vi "VLC Main Open Camera.vi"(11 "Camera 1":refnum<k24>(container)) -> ()   [LabVIEW 2017]
uses:
  System.Windows.Forms
panel:
  in  "Camera 3":refnum<vi>
  in  "path in":path=path "C:/Program Files (x86)/VideoLAN/VLC/libvlc.dll"
  in  "stop":bool
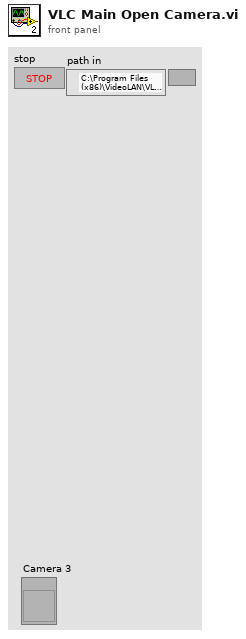
[diagram p1: front panel]
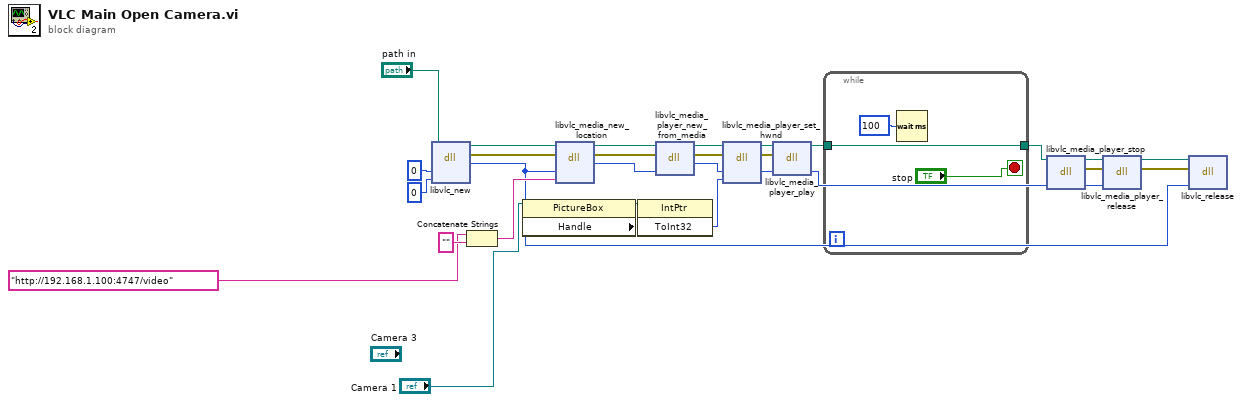
[diagram p0: block diagram]
diagram:
  n1 = dll-call lib="C:/Program Files (x86)/VideoLAN/VLC/libvlc.dll" fn="libvlc_new"(path in="path in", "argc"=i16 0, "argv"=u8 0) -> (path out=w24:path, error out=w21:errorcluster, "return type"=w10:i32)  [unwired: 4 in]
  n2 = Concatenate Strings("http://192.168.1.100:4747/video", "" ("string")) -> (w14:string)
  n3 = property class="PictureBox"(reference="Camera 1") -> ("Handle"=w28:refnum<k24>)  [unwired: 1 in, 2 out]
  n4 = dll-call lib="C:/Program Files (x86)/VideoLAN/VLC/libvlc.dll" fn="libvlc_media_new_location"(path in=w24, error in=w21, "p_instance"=w10, "path"=w14) -> (path out=w27:path, error out=w15:errorcluster, "return type"=w16:i32)  [unwired: 3 in]
  n5 = invoke class="IntPtr" method="ToInt32"(reference=w28) -> ("ToInt32"=w29:i32)  [unwired: 2 in, 2 out]
  n6 = dll-call lib="C:/Program Files (x86)/VideoLAN/VLC/libvlc.dll" fn="libvlc_media_player_new_from_media"(path in=w27, error in=w15, "p_md"=w16) -> (path out=w25:path, error out=w18:errorcluster, "return type"=w20:i32)  [unwired: 2 in]
  n7 = dll-call lib="C:/Program Files (x86)/VideoLAN/VLC/libvlc.dll" fn="libvlc_media_player_set_hwnd"(path in=w25, error in=w18, "p_mi"=w20, "drawable"=w29) -> (path out=w26:path, error out=w17:errorcluster, "p_mi"=w19:i32)  [unwired: 3 in]
  n8 = dll-call lib="C:/Program Files (x86)/VideoLAN/VLC/libvlc.dll" fn="libvlc_media_player_play"(path in=w26, error in=w17, "p_mi"=w19) -> (path out=w4:path, "p_mi"=w11:i32)  [unwired: 2 in, 1 out]
  n9 = while {
    tunnel: w4 -> [w31]
    tunnel: [w31] -> w3
    stop <- "stop" stop-if-true
    n10 = Wait (ms)(milliseconds to wait=u32 100) -> ()  [unwired: 1 out]
  }
  n11 = dll-call lib="C:/Program Files (x86)/VideoLAN/VLC/libvlc.dll" fn="libvlc_media_player_stop"(path in=w3, "p_mi"=w11) -> (path out=w8:path, error out=w5:errorcluster, "p_mi"=w6:i32)  [unwired: 3 in]
  n12 = dll-call lib="C:/Program Files (x86)/VideoLAN/VLC/libvlc.dll" fn="libvlc_media_player_release"(path in=w8, error in=w5, "p_mi"=w6) -> (path out=w9:path, error out=w7:errorcluster)  [unwired: 3 in]
  n13 = dll-call lib="C:/Program Files (x86)/VideoLAN/VLC/libvlc.dll" fn="libvlc_release"(path in=w9, error in=w7, "p_instnace"=w10) -> ()  [unwired: 3 in, 2 out]
